vi "Error Converter (ErrCode or Status).vi"(8 "error in (no error)":errorcluster, 11 "error code":u32) -> (0 "error out":errorcluster)   [LabVIEW 2015, in "AduHid.lvlib"]
uses:
  AduHid.lvlib
  Windows/SysWOW64/kernel32.dll
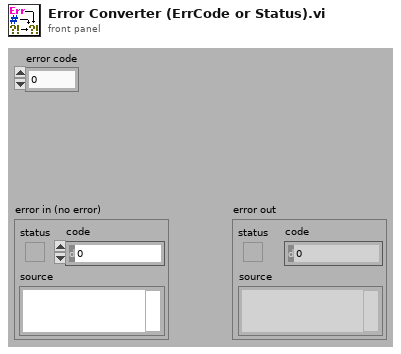
[diagram p1: front panel]
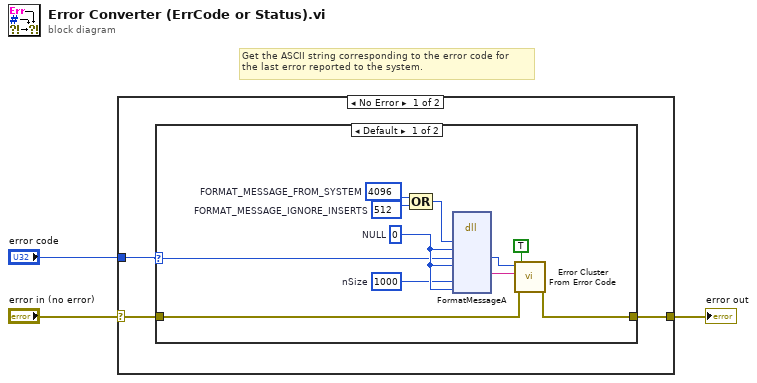
[diagram p0: block diagram]
diagram:
  # "Get the ASCII string corresponding to the error code for\nthe last error reported to the system."
  n1 = case shown="No Error" "error in (no error)" {
    selector: "error in (no error)" -> [w6 w19]
    tunnel: [w5 w19] -> w3
    tunnel: "error code" -> [w4 _]
    frame No Error {
      n2 = case shown="Default" w4 {
        selector: w4 -> [w7 _]
        tunnel: w6 -> [w8 w18]
        tunnel: [w17 w18] -> w5
        frame Default {
          w10 = u32 4096  # FORMAT_MESSAGE_FROM_SYSTEM
          w11 = u32 1000  # nSize
          w14 = u32 512  # FORMAT_MESSAGE_IGNORE_INSERTS
          w12 = u32 0  # NULL
          n3 = Compound Arithmetic op=OR(w10, w14) -> (w13:u32)
          n4 = dll-call lib="C:/Windows/SysWOW64/kernel32.dll" fn="FormatMessageA"("dwFlags"=w13, "lpSource"=w12, "dwMessageId"=w7, "dwLanguageId"=w12, "nSize"=w11, "Arguments"=w12) -> ("dwMessageId"=w9:u32, "lpBuffer"=w15:string)  [unwired: 10 in, 2 out]
          n5 = call <vilib>:"Error Cluster From Error Code.vi"("show call chain? (False)"=TRUE, "error in (no error)"=w8, "error message (\"\")"=w15, "error code (0)"=w9) -> ("error out"=w17:errorcluster)  [unwired: 5 in]
        }
        frame 0 {
        }
      }
    }
    frame Error {
    }
  }
  "error out" <- w3
